vi "Practica 5 Laboratorio.vi"() -> ()   [LabVIEW 2020]
panel:
  in  "Boolean 3":bool=TRUE
  in  "Boolean 2":bool=TRUE
  in  "Boolean":bool=TRUE
  in  "Steer Wheel":i16(slide) scale=-32768.0..32767.0
  in  "stop 2":bool
  in  "stop":bool
  out "Percentage Brake":dbl
  in  "Brake":i16(slide) scale=-32768.0..32767.0
  in  "Gas":i16(slide) scale=-32768.0..32767.0
  out "Dial":dbl(knob) min=0.0 max=900.0 step=1.0 scale=0.0..360.0
  in  "Knob":dbl(knob) scale=0.0..10.0
  out "Fuel \n   L":dbl(knob) scale=0.0..50.0
  out "Temperature\n         5":dbl(knob) scale=0.0..250.0
  out "String":string
  out "D":bool
  out "N":bool
  out "R":bool
  out "P":bool
  out "Meter 2":dbl(knob) scale=-45.0..45.0
  out "Gauge":dbl(knob) scale=0.0..8.0
  out "Gauge 2":dbl(knob) scale=0.0..200.0
  out "Km":dbl
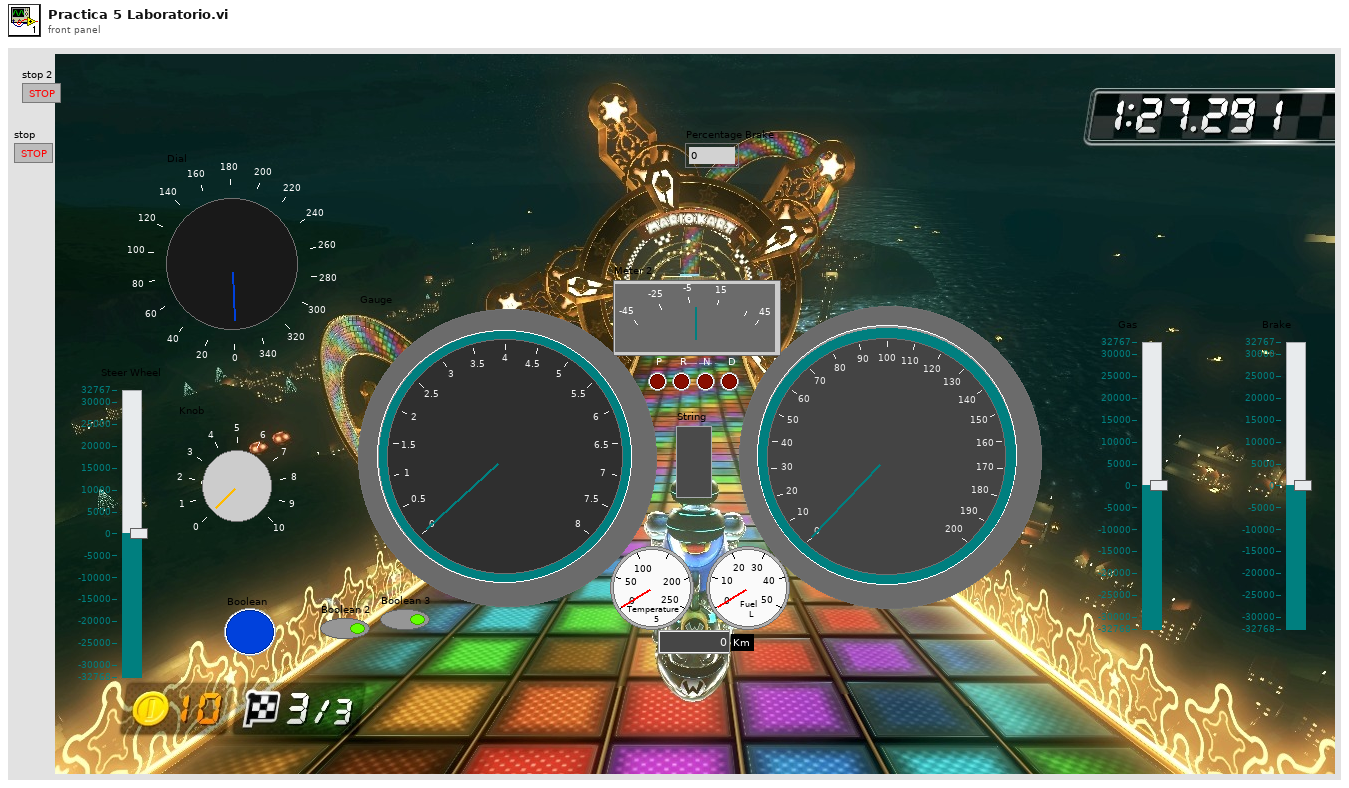
[diagram p1: front panel]
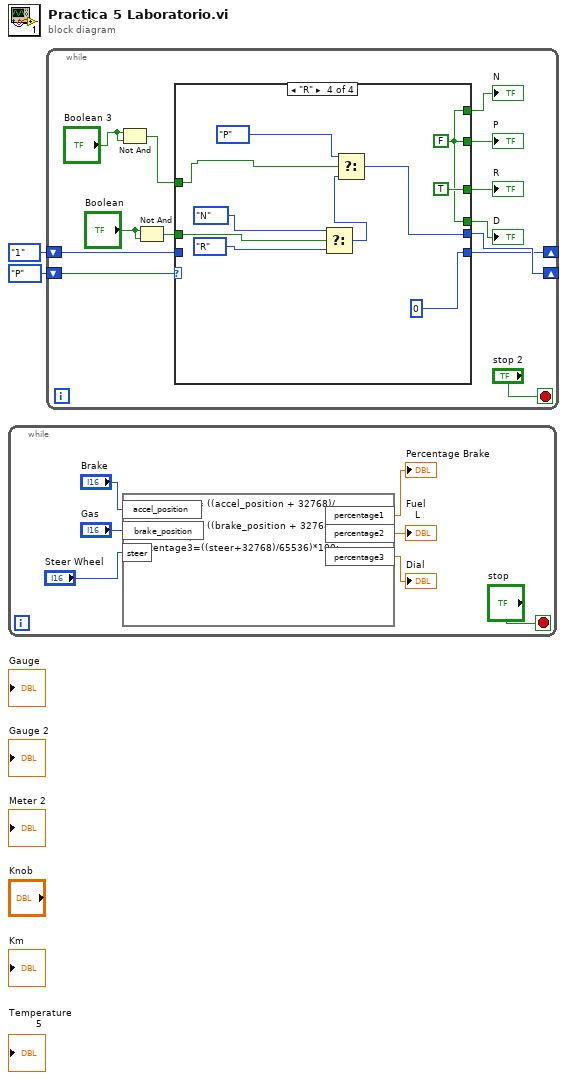
[diagram p0: block diagram]
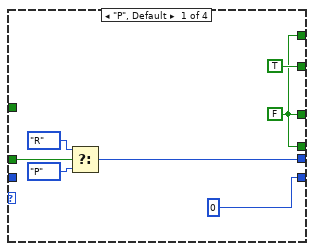
[diagram p2: hidden frame]
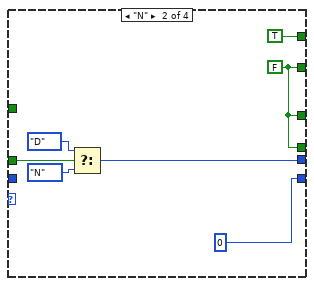
[diagram p3: hidden frame]
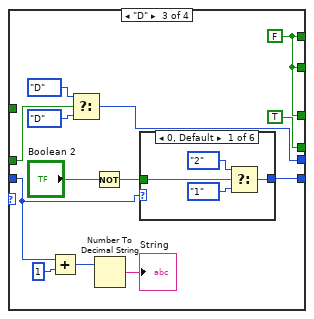
[diagram p4: hidden frame]
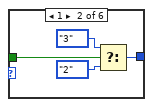
[diagram p5: hidden frame]
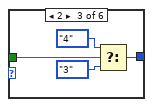
[diagram p6: hidden frame]
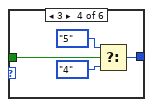
[diagram p7: hidden frame]
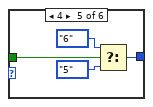
[diagram p8: hidden frame]
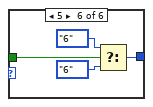
[diagram p9: hidden frame]
diagram:
  n1 = while {
    stop <- "stop" stop-if-true
    n2 = formula code="percentage1 = ((accel_position + 32768)/65536)*100;\npercentage2 = ((brake_position + 32768)/65536)*100;\npercentage3=((steer+32768)/65536)*100;"("accel_position"="Brake", "brake_position"="Gas", "steer"="Steer Wheel") -> ("percentage1"=→"Percentage Brake":dbl, "percentage2"=→"Fuel \n   L":dbl, "percentage3"=→"Dial":dbl)
  }
  n3 = while {
    shift-right: [w20] -> _
    shift-left: enum16{"P", "R", "N", "D", ""}."P" -> [w21]
    shift-right: [w12] -> _
    shift-left: enum16{"1", "2", "3", "4", "5", "6"}."1" -> [w13]
    stop <- "stop 2" stop-if-true
    n4 = Not And(1:"Boolean 3", 2:"Boolean 3") -> (0:w11:bool)
    n5 = Not And(1:"Boolean", 2:"Boolean") -> (0:w14:bool)
    n6 = case shown="\"R\"" w21 {
      tunnel: [w25 w32 w49 w74] -> w20
      tunnel: [TRUE w35 w45 w82] -> w19
      tunnel: [w28 TRUE w45 w82] -> w18
      tunnel: [w28 w35 TRUE w82] -> w17
      tunnel: [w28 w35 w45 TRUE] -> w16
      tunnel: w14 -> [w24 w31 w46 w79]
      tunnel: w13 -> [_ _ w38 _]
      tunnel: [0 0 w37 0] -> w12
      tunnel: w11 -> [_ _ _ w77]
      frame "P", Default {
        w28 = FALSE
        n7 = Select(t=enum16{"P", "R", "N", "D", ""}."R", s=w24, f=enum16{"P", "R", "N", "D", ""}."P") -> (s? t:f=w25:enum16{"P", "R", "N", "D", ""})
      }
      frame "N" {
        w35 = FALSE
        n8 = Select(t=enum16{"P", "R", "N", "D", ""}."D", s=w31, f=enum16{"P", "R", "N", "D", ""}."N") -> (s? t:f=w32:enum16{"P", "R", "N", "D", ""})
      }
      frame "D" {
        w45 = FALSE
        n9 = Add(x=w38, y=1) -> (x+y=w40:i32)
        n10 = Select(t=enum16{"P", "R", "N", "D", ""}."D", s=w46, f=enum16{"P", "R", "N", "D", ""}."D") -> (s? t:f=w49:enum16{"P", "R", "N", "D", ""})
        n11 = Not(x="Boolean 2") -> (.not. x?=w42:bool)
        n12 = Number To Decimal String(number=w40) -> (decimal integer string=→"String":string)  [unwired: 1 in]
        n13 = case shown="0, Default" w38 {
          tunnel: w42 -> [w52 w54 w58 w62 w66 w70]
          tunnel: [w53 w57 w61 w65 w69 w73] -> w37
          frame 0, Default {
            n14 = Select(t=enum16{"1", "2", "3", "4", "5", "6"}."2", s=w52, f=enum16{"1", "2", "3", "4", "5", "6"}."1") -> (s? t:f=w53:enum16{"1", "2", "3", "4", "5", "6"})
          }
          frame 1 {
            n15 = Select(t=enum16{"1", "2", "3", "4", "5", "6"}."3", s=w54, f=enum16{"1", "2", "3", "4", "5", "6"}."2") -> (s? t:f=w57:enum16{"1", "2", "3", "4", "5", "6"})
          }
          frame 2 {
            n16 = Select(t=enum16{"1", "2", "3", "4", "5", "6"}."4", s=w58, f=enum16{"1", "2", "3", "4", "5", "6"}."3") -> (s? t:f=w61:enum16{"1", "2", "3", "4", "5", "6"})
          }
          frame 3 {
            n17 = Select(t=enum16{"1", "2", "3", "4", "5", "6"}."5", s=w62, f=enum16{"1", "2", "3", "4", "5", "6"}."4") -> (s? t:f=w65:enum16{"1", "2", "3", "4", "5", "6"})
          }
          frame 4 {
            n18 = Select(t=enum16{"1", "2", "3", "4", "5", "6"}."6", s=w66, f=enum16{"1", "2", "3", "4", "5", "6"}."5") -> (s? t:f=w69:enum16{"1", "2", "3", "4", "5", "6"})
          }
          frame 5 {
            n19 = Select(t=enum16{"1", "2", "3", "4", "5", "6"}."6", s=w70, f=enum16{"1", "2", "3", "4", "5", "6"}."6") -> (s? t:f=w73:enum16{"1", "2", "3", "4", "5", "6"})
          }
        }
      }
      frame "R" {
        w82 = FALSE
        n20 = Select(t=enum16{"P", "R", "N", "D", ""}."N", s=w79, f=enum16{"P", "R", "N", "D", ""}."R") -> (s? t:f=w75:enum16{"P", "R", "N", "D", ""})
        n21 = Select(t=enum16{"P", "R", "N", "D", ""}."P", s=w77, f=w75) -> (s? t:f=w74:enum16{"P", "R", "N", "D", ""})
      }
    }
    "P" <- w19
    "R" <- w16
    "D" <- w17
    "N" <- w18
  }
